vi "LD Monitor.vi"() -> ()   [LabVIEW 2017]
uses:
  <vilib>/Utility/error.llb/Clear Errors.vi
  <instrlib>/tio-labview/TIO Library/Data Stream/TIO Data Stream Parse Description.vi
panel:
  in  "Save":bool
  in  "Autostart":bool
  in  "TEC Current Limit":dbl[unit]=0.1
  out "Kill":bool=TRUE
  in  "Max Current":dbl[unit]=0.1
  in  "Current":dbl[unit]=0.1
  in  "Temperature":dbl[unit]=100.0
  in  "Current Enable":bool
  in  "TEC Enable":bool
  in  "URL":refnum<visa-resource-name>="tcp://localhost"
  out "ID":string
  in  "Quit":bool
  in  "Duration":dbl[unit]=100.0
  in  "Reset":bool
  out "Temperature":cluster{dbl, dbl, dbl[]}(graph)={407.109653, 0.002, []}
  out "TEC":cluster{dbl, dbl, dbl[]}(graph)={407.109653, 0.002, []}
  # "Laser Driver"
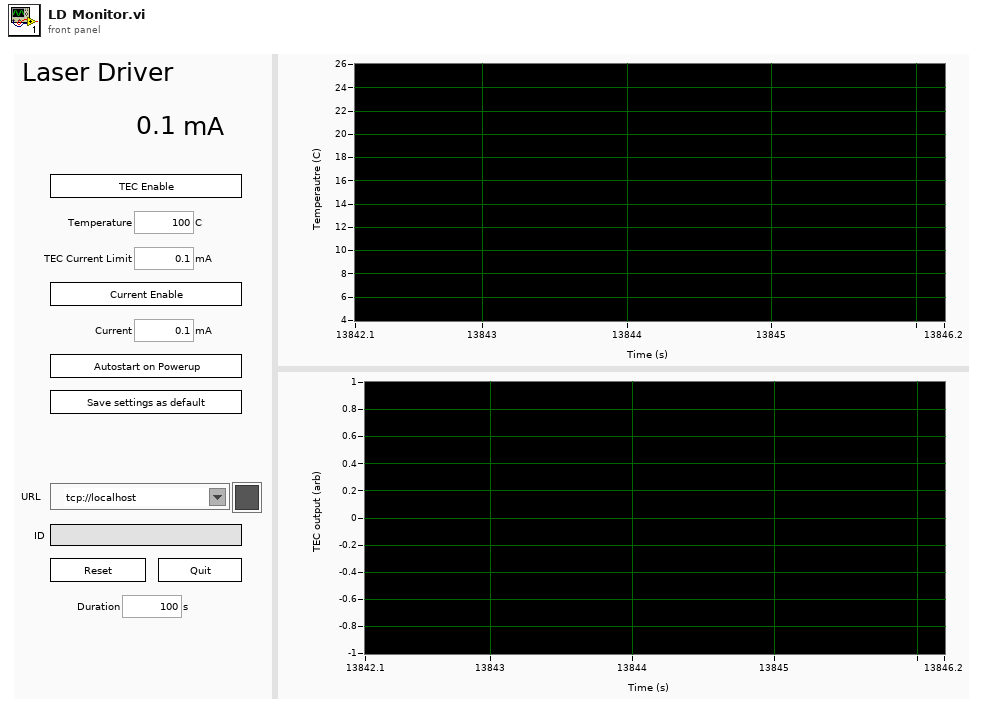
[diagram p1: front panel]
types:
  T1 = cluster{"Type":enum16{"TCP", "Serial"}, "Serial":refnum<visa-resource-name>, "TCP":refnum<k5>, "Timeout":u32}
  T2 = cluster{"Stream Description":cluster{"Stream ID":u16, "Data Type":u8, "Channels":u8, "Restart ID":u16, "Start timestamp (s)":dbl, "Sample counter":u64, "Period (s)":dbl, "Flags":u8, "Timestamp type":u8, "Name":string, "Last sample number":u64, "Last Restart ID":u16, "Version":u16, "Sample Size":u16}, "Sample #":u32, "Raw Data":string}
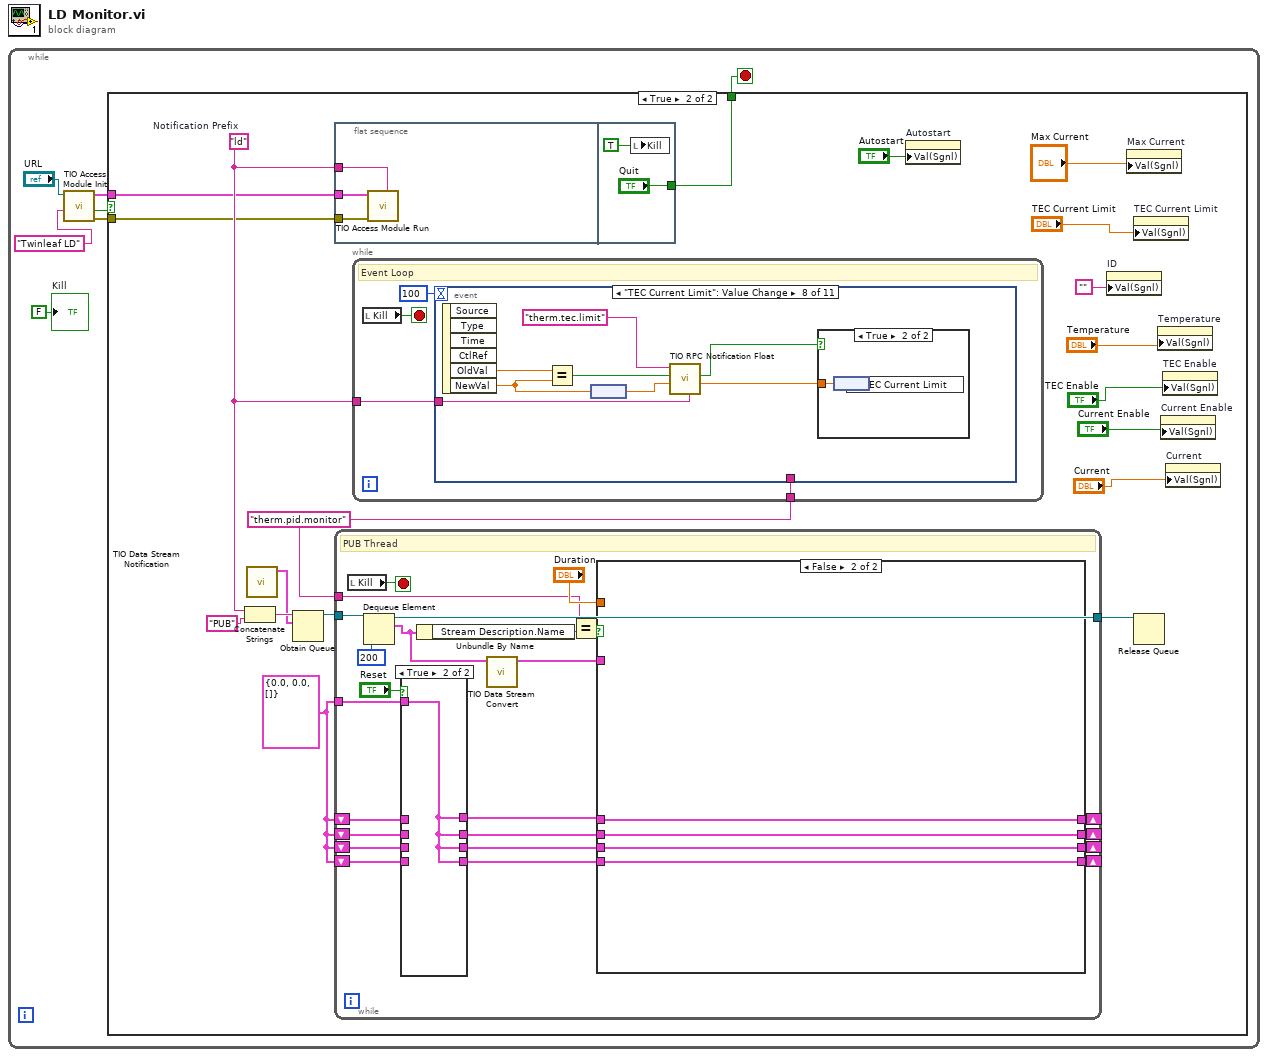
[diagram p0: block diagram]
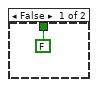
[diagram p2: hidden frame]
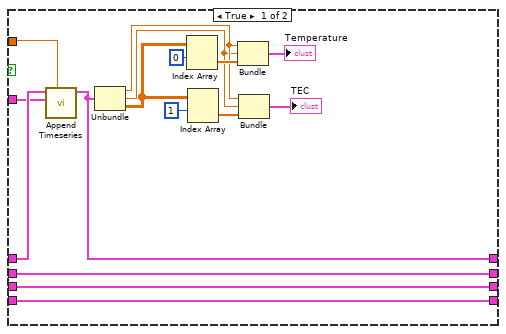
[diagram p4: hidden frame]
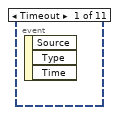
[diagram p5: hidden frame]
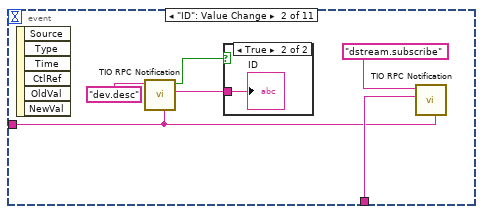
[diagram p6: hidden frame]
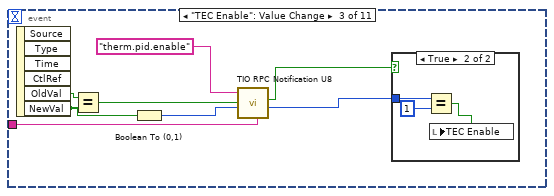
[diagram p8: hidden frame]
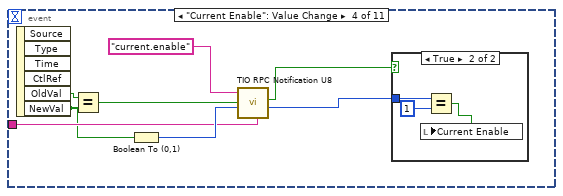
[diagram p10: hidden frame]
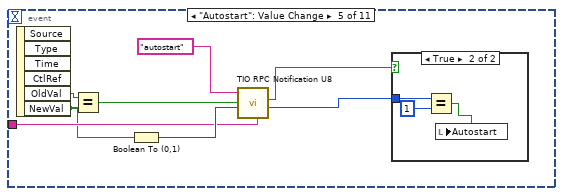
[diagram p12: hidden frame]
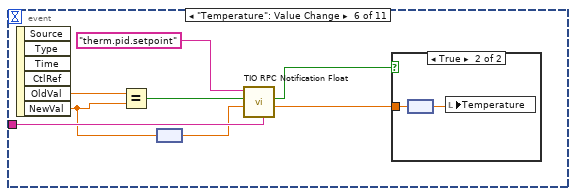
[diagram p14: hidden frame]
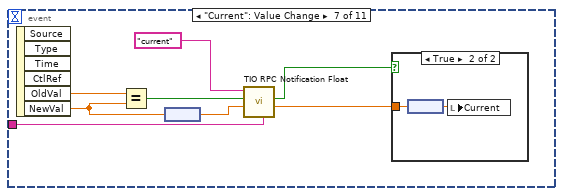
[diagram p16: hidden frame]
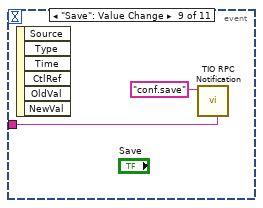
[diagram p19: hidden frame]
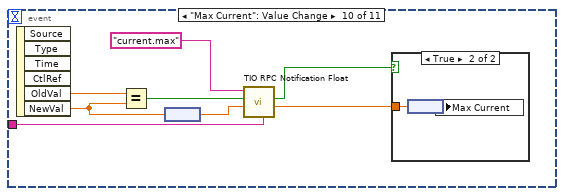
[diagram p20: hidden frame]
diagram:
  n1 = while {
    stop <- w2 stop-if-true
    n2 = call <instrlib>:"TIO Access Module Init.vi"("ID"="Twinleaf LD" ("Prefix"), "URL"="URL") -> ("error out"=w4:errorcluster, "Connected"=w3:bool, "TS Connection"=w5:T1)  [unwired: 7 in]
    n3 = case shown="True" w3 {
      tunnel: w5 -> [_ w19]
      tunnel: w4 -> [_ w18]
      tunnel: [FALSE ("Quit") w17] -> w2
      frame False {
      }
      frame True {
        w16 = "therm.pid.monitor" ("name (unnamed)")
        w20 = "ld"  # Notification Prefix
        w22 = cluster{dbl, dbl, dbl[][]} {0.0, 0.0, []} ("Waveform Timeseries")
        n4 = Concatenate Strings(w20, "PUB" ("name (unnamed)")) -> (w26:string)
        n5 = call <instrlib>:"TIO Data Stream Notification.vi"() -> ("Data Stream Notification"=w21:T2)  [unwired: 11 in]
        n6 = Obtain Queue(name (unnamed)=w26, element data type=w21) -> (queue out=w24:refnum<queue>)  [unwired: 3 in, 2 out]
        n7 = flat-sequence {
          tunnel: w20 -> [w77]
          tunnel: w19 -> [w79]
          tunnel: w18 -> [w78]
          tunnel: ["Quit"] -> w17
          frame #0 {
            n8 = call <instrlib>:"TIO Access Module Run.vi"("Notification Prefix"=w77, "error in (no error)"=w78, "TS Connection"=w79) -> ()  [unwired: 9 in]
          }
          frame #1 {
            n9 = local write "Kill"(TRUE ("Kill")) -> ()
          }
        }
        n10 = while {
          tunnel: w24 -> [w49]
          shift-right: [w48] -> _
          shift-left: w22 -> [w46]
          tunnel: w22 -> [w45]
          shift-right: [w42] -> _
          shift-left: w22 -> [w41]
          shift-right: [w39] -> _
          shift-left: w22 -> [w37]
          tunnel: [w36] -> w23
          shift-right: [w34] -> _
          shift-left: w22 -> [w35]
          tunnel: w16 -> [w28]
          stop <- w50 stop-if-true
          # "PUB Thread"
          n11 = local read "Kill"() -> (w50:bool)
          n12 = Dequeue Element(queue=w49, timeout in ms (-1)=200) -> (queue out=w36:refnum<queue>, element=w31:T2)  [unwired: 1 in, 2 out]
          n13 = case shown="True" "Reset" {
            tunnel: w46 -> [w55 _]
            tunnel: [w55 w56] -> w44
            tunnel: w45 -> [_ w56]
            tunnel: w41 -> [w54 _]
            tunnel: [w54 w56] -> w40
            tunnel: [w53 w56] -> w38
            tunnel: w37 -> [w53 _]
            tunnel: [w52 w56] -> w33
            tunnel: w35 -> [w52 _]
            frame False {
            }
            frame True {
            }
          }
          n14 = Unbundle By Name(w31) -> ("Stream Description.Name"=w30:string)
          n15 = call <instrlib>:"TIO Data Stream Convert.vi"("Data Stream Notification"=w31) -> ("Waveform"=w32:cluster{dbl, dbl, dbl[][]})  [unwired: 10 in]
          n16 = Equal?(x=w28, y=w30) -> (x = y?=w29:bool)
          n17 = case shown="False" w29 {
            tunnel: "Duration" -> [w72 _]
            tunnel: [w70 w76] -> w48
            tunnel: w44 -> [w69 w76]
            tunnel: [w67 w75] -> w42
            tunnel: w40 -> [w67 w75]
            tunnel: [w66 w74] -> w39
            tunnel: w38 -> [w66 w74]
            tunnel: [w64 w73] -> w34
            tunnel: w33 -> [w64 w73]
            tunnel: w32 -> [w63 _]
            frame True {
              n18 = call <instrlib>:"Append Timeseries.vi"("Duration"=w72, "Waveform New"=w63, "Waveform History"=w69) -> ("Waveform Timeseries"=w70:cluster{dbl, dbl, dbl[][]})  [unwired: 8 in]
              n19 = Unbundle(w70) -> (w61:dbl, w60:dbl, w59:dbl[][])
              n20 = Index Array(array=w59, index (row)=0 ("disabled index (col)")) -> (element=w68:dbl[])  [unwired: 1 in]
              n21 = Index Array(array=w59, index (row)=1) -> (element=w62:dbl[])  [unwired: 1 in]
              n22 = Bundle(w61, w60, w68) -> (→"Temperature":cluster{dbl, dbl, dbl[]})  [unwired: 1 in]
              n23 = Bundle(w61, w60, w62) -> (→"TEC":cluster{dbl, dbl, dbl[]})  [unwired: 1 in]
            }
            frame False {
            }
          }
        }
        n24 = while {
          tunnel: w20 -> [w83]
          tunnel: w16 -> [w82]
          stop <- w85 stop-if-true
          # "Event Loop"
          n25 = local read "Kill"() -> (w85:bool)
          n26 = event shown="[7] \"TEC Current Limit\": Value Change" {
            selector: _ -> [_ _ _ _ _ _ _ _ _ _ _]
            dyn-events: _ -> [_ _ _ _ _ _ _ _ _ _ _]
            timeout: 100 -> [_ _ _ _ _ _ _ _ _ _ _]
            tunnel: w83 -> [_ w86 w96 w107 w118 w131 w141 w151 w157 w163 w168]
            tunnel: w82 -> [_ w87 _ _ _ _ _ _ _ _ w169]
            event Timeout {
              n27 = event-data() -> ()  [unwired: 1 in, 3 out]
            }
            event "ID": Value Change {
              n28 = event-data() -> ()  [unwired: 1 in, 6 out]
              n29 = call <instrlib>:"TIO RPC Notification.vi"("Notification Prefix"=w86, "Topic"="dev.desc") -> ("REP"=w90:string, "Response"=w89:bool)  [unwired: 6 in, 1 out]
              n30 = case shown="True" w89 {
                tunnel: w90 -> [_ w92]
                frame False {
                }
                frame True {
                  "ID" <- w92
                }
              }
              n31 = call <instrlib>:"TIO RPC Notification.vi"("Notification Prefix"=w86, "Payload"=w87, "Topic"="dstream.subscribe") -> ()  [unwired: 5 in, 3 out]
            }
            event "TEC Enable": Value Change {
              n32 = event-data() -> ("OldVal"=w99:bool, "NewVal"=w93:bool)  [unwired: 1 in, 4 out]
              n33 = Equal?(x=w99, y=w93) -> (x = y?=w98:bool)
              n34 = Boolean To (0,1)(Boolean=w93) -> (0, 1=w97:i16)
              n35 = call <instrlib>:"TIO RPC Notification U8.vi"("Notification Prefix"=w96, "U8"=w97, "Read"=w98, "String"="therm.pid.enable" ("Topic")) -> ("U8"=w94:u8, "Response"=w95:bool)  [unwired: 4 in, 1 out]
              n36 = case shown="True" w95 {
                tunnel: w94 -> [_ w103]
                frame False {
                }
                frame True {
                  n37 = Equal?(x=w103, y=u8 1) -> (x = y?=w101:bool)
                  n38 = local write "TEC Enable"(w101) -> ()
                }
              }
            }
            event "Current Enable": Value Change {
              n39 = event-data() -> ("OldVal"=w110:bool, "NewVal"=w104:bool)  [unwired: 1 in, 4 out]
              n40 = Equal?(x=w110, y=w104) -> (x = y?=w109:bool)
              n41 = Boolean To (0,1)(Boolean=w104) -> (0, 1=w108:i16)
              n42 = call <instrlib>:"TIO RPC Notification U8.vi"("Notification Prefix"=w107, "U8"=w108, "Read"=w109, "String"="current.enable" ("Topic")) -> ("U8"=w105:u8, "Response"=w106:bool)  [unwired: 4 in, 1 out]
              n43 = case shown="True" w106 {
                tunnel: w105 -> [_ w114]
                frame False {
                }
                frame True {
                  n44 = Equal?(x=w114, y=u8 1) -> (x = y?=w112:bool)
                  n45 = local write "Current Enable"(w112) -> ()
                }
              }
            }
            event "Autostart": Value Change {
              n46 = event-data() -> ("OldVal"=w121:bool, "NewVal"=w115:bool)  [unwired: 1 in, 4 out]
              n47 = Equal?(x=w121, y=w115) -> (x = y?=w120:bool)
              n48 = Boolean To (0,1)(Boolean=w115) -> (0, 1=w119:i16)
              n49 = call <instrlib>:"TIO RPC Notification U8.vi"("Notification Prefix"=w118, "U8"=w119, "Read"=w120, "String"="autostart" ("Topic")) -> ("U8"=w116:u8, "Response"=w117:bool)  [unwired: 4 in, 1 out]
              n50 = case shown="True" w117 {
                tunnel: w116 -> [_ w125]
                frame False {
                }
                frame True {
                  n51 = Equal?(x=w125, y=u8 1) -> (x = y?=w123:bool)
                  n52 = local write "Autostart"(w123) -> ()
                }
              }
            }
            event "Temperature": Value Change {
              n53 = event-data() -> ("OldVal"=w127:dbl[unit], "NewVal"=w126:dbl[unit])  [unwired: 1 in, 4 out]
              n54 = Equal?(x=w127, y=w126) -> (x = y?=w132:bool)
              n55 = node(w126) -> (w130:dbl)
              n56 = call <instrlib>:"TIO RPC Notification Float.vi"("Notification"=w131, "Set value"=w130, "Read"=w132, "String"="therm.pid.setpoint" ("Topic")) -> ("Get value (default if error)"=w129:sgl, "Response"=w128:bool)  [unwired: 4 in, 1 out]
              n57 = case shown="True" w128 {
                tunnel: w129 -> [_ w135]
                frame False {
                }
                frame True {
                  n58 = node(w135) -> (w134:sgl[unit])
                  n59 = local write "Temperature"(w134) -> ()
                }
              }
            }
            event "Current": Value Change {
              n60 = event-data() -> ("OldVal"=w137:dbl[unit], "NewVal"=w136:dbl[unit])  [unwired: 1 in, 4 out]
              n61 = Equal?(x=w137, y=w136) -> (x = y?=w142:bool)
              n62 = node(w136) -> (w140:dbl)
              n63 = call <instrlib>:"TIO RPC Notification Float.vi"("Notification"=w141, "Set value"=w140, "Read"=w142, "String"="current" ("Topic")) -> ("Get value (default if error)"=w139:sgl, "Response"=w138:bool)  [unwired: 4 in, 1 out]
              n64 = case shown="True" w138 {
                tunnel: w139 -> [_ w145]
                frame False {
                }
                frame True {
                  n65 = node(w145) -> (w144:sgl[unit])
                  n66 = local write "Current"(w144) -> ()
                }
              }
            }
            event "TEC Current Limit": Value Change {
              n67 = event-data() -> ("OldVal"=w147:dbl[unit], "NewVal"=w146:dbl[unit])  [unwired: 1 in, 4 out]
              n68 = Equal?(x=w147, y=w146) -> (x = y?=w152:bool)
              n69 = node(w146) -> (w150:dbl)
              n70 = call <instrlib>:"TIO RPC Notification Float.vi"("Notification"=w151, "Set value"=w150, "Read"=w152, "String"="therm.tec.limit" ("Topic")) -> ("Get value (default if error)"=w149:sgl, "Response"=w148:bool)  [unwired: 4 in, 1 out]
              n71 = case shown="True" w148 {
                tunnel: w149 -> [_ w155]
                frame False {
                }
                frame True {
                  n72 = node(w155) -> (w154:sgl[unit])
                  n73 = local write "TEC Current Limit"(w154) -> ()
                }
              }
            }
            event "Save": Value Change {
              n74 = event-data() -> ()  [unwired: 1 in, 6 out]
              n75 = call <instrlib>:"TIO RPC Notification.vi"("Notification Prefix"=w157, "Topic"="conf.save") -> ()  [unwired: 6 in, 3 out]
            }
            event "Max Current": Value Change {
              n76 = event-data() -> ("OldVal"=w159:dbl[unit], "NewVal"=w158:dbl[unit])  [unwired: 1 in, 4 out]
              n77 = Equal?(x=w159, y=w158) -> (x = y?=w164:bool)
              n78 = node(w158) -> (w162:dbl)
              n79 = call <instrlib>:"TIO RPC Notification Float.vi"("Notification"=w163, "Set value"=w162, "Read"=w164, "String"="current.max" ("Topic")) -> ("Get value (default if error)"=w161:sgl, "Response"=w160:bool)  [unwired: 4 in, 1 out]
              n80 = case shown="True" w160 {
                tunnel: w161 -> [_ w167]
                frame False {
                }
                frame True {
                  n81 = node(w167) -> (w166:sgl[unit])
                  n82 = local write "Max Current"(w166) -> ()
                }
              }
            }
            event "Quit": Value Change {
              n83 = event-data() -> ("NewVal"=w171:bool)  [unwired: 1 in, 5 out]
              n84 = call <instrlib>:"TIO RPC Notification.vi"("Notification Prefix"=w168, "Payload"=w169, "Topic"="dstream.unsubscribe") -> ()  [unwired: 5 in, 3 out]
              n85 = case shown="True" w171 {
                tunnel: w168 -> [_ w172]
                frame False {
                }
                frame True {
                  w173 = TRUE ("Kill")
                  n86 = Concatenate Strings(w172, "QUIT" ("name (unnamed)")) -> (w178:string)
                  n87 = Obtain Notifier(name (unnamed)=w178, notification data type=FALSE ("Connected")) -> (notifier out=w175:refnum<notifier>, error out=w176:errorcluster)  [unwired: 2 in, 1 out]
                  n88 = Send Notification(notification=w173, notifier=w175, error in (no error)=w176) -> ()  [unwired: 2 out]
                  n89 = local write "Kill"(w173) -> ()
                }
              }
            }
          }
        }
        n90 = property on="Autostart" class="Bool (strict)"("Val(Sgnl)"="Autostart") -> ()  [unwired: 2 in, 2 out]
        n91 = property on="ID" class="Str"("Val(Sgnl)"="") -> ()  [unwired: 2 in, 2 out]
        n92 = property on="Max Current" class="DigNum (strict)"("Val(Sgnl)"="Max Current") -> ()  [unwired: 2 in, 2 out]
        n93 = property on="TEC Current Limit" class="DigNum (strict)"("Val(Sgnl)"="TEC Current Limit") -> ()  [unwired: 2 in, 2 out]
        n94 = Release Queue(queue=w23) -> ()  [unwired: 2 in, 3 out]
        n95 = property on="Temperature" class="DigNum (strict)"("Val(Sgnl)"="Temperature") -> ()  [unwired: 2 in, 2 out]
        n96 = property on="Current Enable" class="Bool (strict)"("Val(Sgnl)"="Current Enable") -> ()  [unwired: 2 in, 2 out]
        n97 = property on="TEC Enable" class="Bool (strict)"("Val(Sgnl)"="TEC Enable") -> ()  [unwired: 2 in, 2 out]
        n98 = property on="Current" class="DigNum (strict)"("Val(Sgnl)"="Current") -> ()  [unwired: 2 in, 2 out]
      }
    }
    "Kill" <- FALSE ("Kill")
  }
